vi "Load Model.vi"(0 "reference in":refnum<class "Battery.lvclass">, 2 "Model Parameters":T1={"chemistry"="Chen2020", "model_type"="SPMe"}, 5 "Error In":errorcluster) -> (14 "reference out":refnum<class "Battery.lvclass">, 16 "model loaded":bool, 19 "Error Out":errorcluster)   [LabVIEW 2023, in "Battery.lvclass"]
uses:
  Battery.lvclass
  Battery.lvclass/Battery.ctl
  Model Parameters.ctl
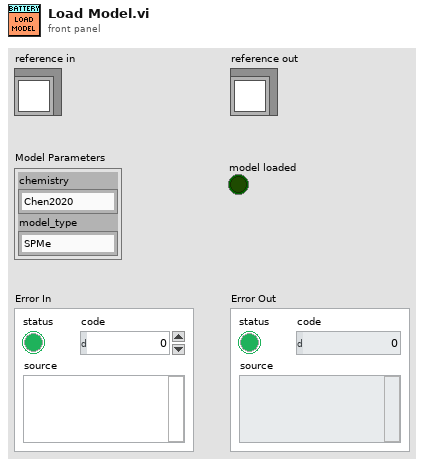
[diagram p1: front panel]
types:
  T1 = typedef "Battery.lvclass/Model Parameters.ctl" = cluster{"chemistry":string, "model_type":string}
  T2 = typedef "Battery.lvclass/ObjectAttributes.ctl" = cluster{"Python module":path, "Python Session":refnum<k35>, "PybammWrapper":refnum<k38>, "model loaded":bool, "simulation loaded":bool, "simulation enabled":bool, "SOC OCV Curve":dbl[][], "Open Circuit Voltage (V)":dbl, "State of Charge (%)":dbl, "# Cells in Series":u16, "# Cells in Parallel":u16, "Model Parameters":T1, "Simulation Parameters":T3, "Power Module":refnum<class "PowerModuleInterface.lvclass">}
  T3 = typedef "Battery.lvclass/Simulation Parameters.ctl" = cluster{"num_rc_pairs":i32, "R0":dbl, "R1":dbl, "C1":dbl, "R2":dbl, "C2":dbl, " nominal_capacity_Ah":dbl, "upper_voltage_cutoff":dbl, "lower_voltage_cutoff":dbl}
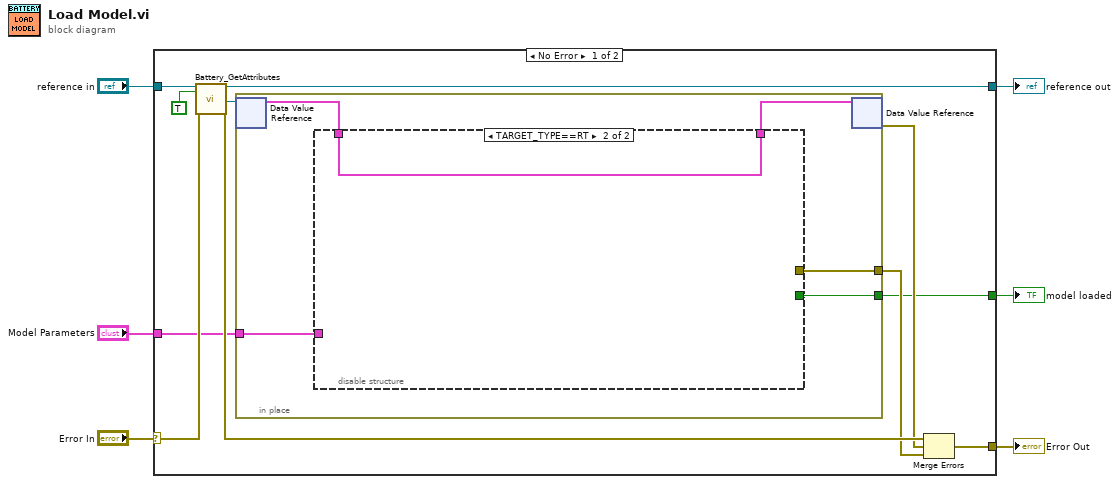
[diagram p0: block diagram]
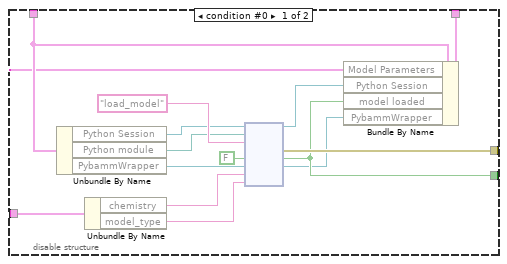
[diagram p2: hidden frame]
diagram:
  n1 = case shown="No Error" "Error In" {
    selector: "Error In" -> [w16 w39]
    tunnel: [w14 w39] -> w5
    tunnel: [w15 w38] -> w3
    tunnel: "reference in" -> [w17 w38]
    tunnel: "Model Parameters" -> [w9 _]
    tunnel: [w7 _] -> w1
    frame No Error {
      n2 = call "Battery_GetAttributes.vi"("reference in"=w17, "OnlyGetDvrReference(False)"=TRUE, "Error In"=w16) -> ("reference out"=w15:refnum<class "Battery.lvclass">, "DataRef"=w13:refnum<data-value>, "Error Out"=w11:errorcluster)  [unwired: 13 in, 1 out]
      n3 = in-place {
        in-place-border: w9 -> [w18]
        in-place-border: [w20] -> w8
        in-place-border: [w19] -> w7
        n4 = in-place-dvr #1(w13) -> (w21:T2)  [unwired: 1 out]
        n5 = disable-structure shown="TARGET_TYPE==RT" {
          disable-tunnel: [w36 w37] -> w22
          disable-tunnel: w21 -> [w35 w37]
          disable-tunnel: [w27 _] -> w20
          disable-tunnel: [w26 _] -> w19
          disable-tunnel: w18 -> [w23 _]
          frame condition #0 {
            n6 = Unbundle By Name(w35) -> ("Python Session"=w29:refnum<k35>, "Python module"=w28:path, "PybammWrapper"=w30:refnum<k38>)
            n7 = Unbundle By Name(w23) -> ("chemistry"=w33:string, "model_type"=w34:string)
            n8 = node(w29, w28, "load_model" ("function name"), FALSE, w30, w33, w34) -> (w24:refnum<k35>, w27:errorcluster, w26:bool, w25:refnum<k38>)  [unwired: 3 in, 2 out]
            n9 = Bundle By Name(cluster=w35, "Model Parameters"=w23, "Python Session"=w24, "model loaded"=w26, "PybammWrapper"=w25) -> (w36:T2)
          }
          frame condition #1 (active) {
          }
        }
        n10 = in-place-dvr #1(w22) -> (w10:errorcluster)  [unwired: 1 out]
      }
      n11 = Merge Errors(w11, w10, w8) -> (w14:errorcluster)
    }
    frame Error {
    }
  }
  "Error Out" <- w5
  "reference out" <- w3
  "model loaded" <- w1
